vi "Build Notifier Controller.vi"(4 "Paras In 2":variant, 6 "Paras In":variant, 7 "Simiple Map Notifier Controller Factory in":refnum<class "Simiple Map Notifier Controller Factory.lvclass">, 8 "error in (no error)":errorcluster, 9 "Notifier Type":refnum<class "Notifier.lvclass">, 10 "System Actors In":refnum<class "System Actor.lvclass">[](array[class]), 11 "Root Actor In":refnum<class "Root Actor.lvclass">) -> (0 "error out":errorcluster, 2 "System Actors Out":refnum<class "System Actor.lvclass">[](array[class]), 3 "Root Actor Out":refnum<class "Root Actor.lvclass">, 5 "Simiple Map Notifier Controller Factory out":refnum<class "Simiple Map Notifier Controller Factory.lvclass">)   [LabVIEW 2024, in "Simiple Map Notifier Controller Factory.lvclass"]
uses:
  Simiple Map Notifier Controller Factory.lvclass
  Ancestor Class/Actor/Root Actor/Root Actor.lvclass
  Ancestor Class/Actor/System Actor/System Actor.lvclass
  Ancestor Class/Actor Assistant/Notifier/Notifier.lvclass
  Notifier Controller/Map Notifier Controller/Map Notifier Controller.lvclass
  C:/Users/iio/Desktop/Bussiness/Tricorn Re/Madelbrot 4.0/General Library/Ancestor Class/Notifier Controller/Notifier Controller.lvclass
  Ancestor Class/Actor/System Actor/System Actor.lvclass/System Actor.ctl
  Simiple Map Notifier Controller Factory.lvclass/Simiple Map Notifier Controller Factory.ctl
  Ancestor Class/Actor/Root Actor/Root Actor.lvclass/Root Actor.ctl
  Ancestor Class/Actor/System Actor/Public Data/Read ID.vi
  Ancestor Class/Actor/System Actor/Public Data/Write Stop Notifier.vi
  Ancestor Class/Actor/Root Actor/Public Data/Write Notifier Controller.vi
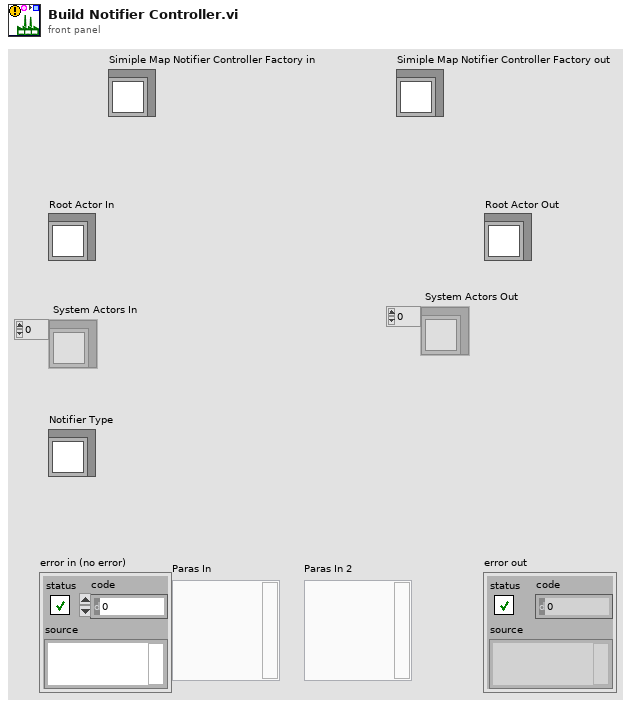
[diagram p1: front panel]
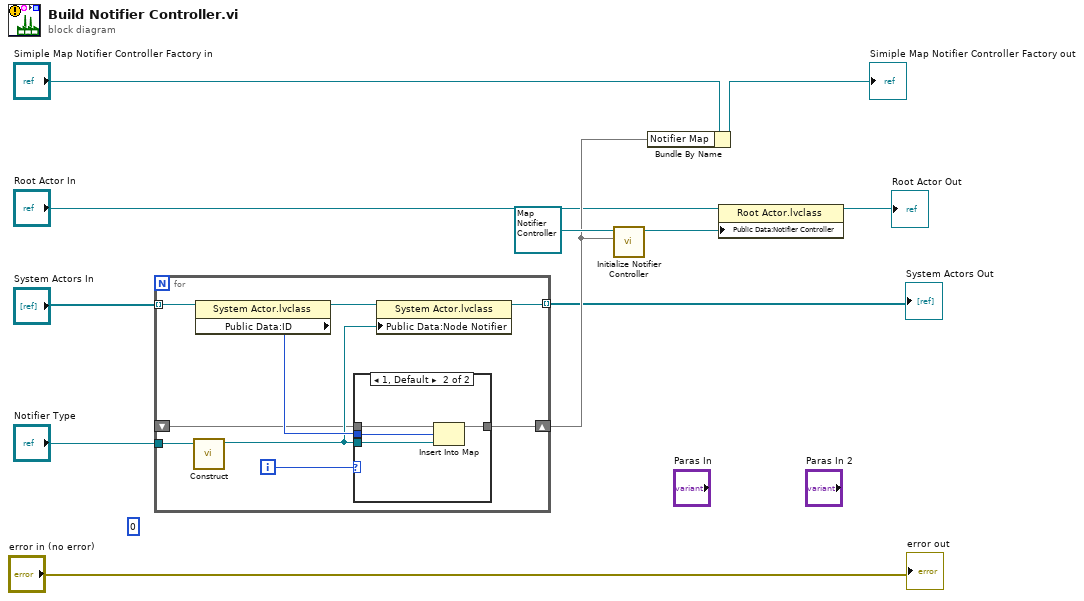
[diagram p0: block diagram]
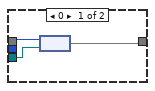
[diagram p2: hidden frame]
diagram:
  (unwired) i64 0 ("ID")
  n1 = for {
    tunnel: "System Actors In" -> [w20] mode=indexing
    shift-right: [w18] -> w8
    shift-left: _ -> [w12]
    tunnel: [w16] -> w2 mode=indexing
    tunnel: "Notifier Type" -> [w14]
    i -> [w13]
    n2 = call-dynamic "Construct.vi"("Notifier in"=w14) -> ("Notifier out"=w15:refnum<class "Notifier.lvclass">)  [unwired: 9 in, 1 out]
    n3 = property class="System Actor.lvclass"(reference=w20) -> (reference out=w17:refnum<class "System Actor.lvclass">, "Public Data:ID"=w19:i64)  [unwired: 1 in, 1 out]
    n4 = case shown="1, Default" w13 {
      tunnel: w19 -> [w23 w27]
      tunnel: [w21 w26] -> w18
      tunnel: w15 -> [w22 w25]
      tunnel: w12 -> [_ w24]
      frame 0 {
        n5 = node(w23, w22) -> (w21:map{i64, refnum<class "Notifier.lvclass">})
      }
      frame 1, Default {
        n6 = Insert Into Map(map in=w24, key=w27, value=w25) -> (map out=w26:map{i64, refnum<class "Notifier.lvclass">})  [unwired: 2 out]
      }
    }
    n7 = property class="System Actor.lvclass"(reference=w17, "Public Data:Node Notifier"=w15) -> (reference out=w16:refnum<class "System Actor.lvclass">)  [unwired: 1 in, 1 out]
  }
  "System Actors Out" <- w2
  n8 = call-dynamic "Initialize Notifier Controller.vi"("Paras In"=w8, "Simple Map Notifier Controller in"=refnum<class "Map Notifier Controller.lvclass"> refnum ("Simple Map SEQ I64 Notifier Controller.lvclass")) -> ("Simple Map Notifier Controller out"=w10:refnum<class "Map Notifier Controller.lvclass">)  [unwired: 8 in, 1 out]
  n9 = Bundle By Name(cluster="Simiple Map Notifier Controller Factory in", "Notifier Map"=w8) -> (→"Simiple Map Notifier Controller Factory out":refnum<class "Simiple Map Notifier Controller Factory.lvclass">)
  n10 = property class="Root Actor.lvclass"(reference="Root Actor In", "Public Data:Notifier Controller"=w10) -> (reference out=→"Root Actor Out":refnum<class "Root Actor.lvclass">)  [unwired: 1 in, 1 out]
  "error out" <- "error in (no error)"
